vi "Vision Research Phantom Series PhFile Error Handler.vi"(0 "Error Code (0)":i32, 5 "Error In (no error)":errorcluster) -> (19 "Error Out":errorcluster)   [LabVIEW 2013, in "VRI.lvlib"]
doc: "This VI calls the PhGetErrorMessage funciton prototype for the PhFile.dll associated with the Vision Research Phantom Series cameras. An error message is created if an error code is returned.\n\nPlace this VI after any PhFile.dll call"
uses:
  VRI.lvlib
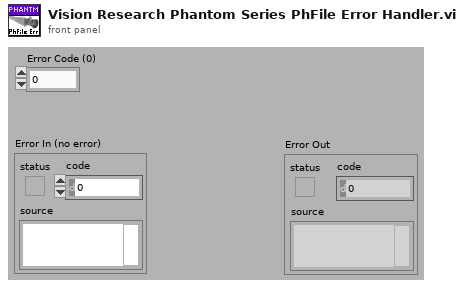
[diagram p1: front panel]
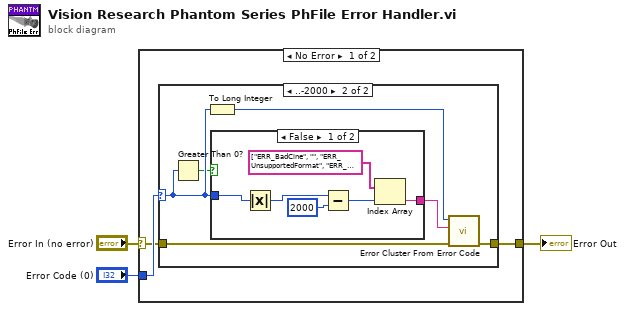
[diagram p0: block diagram]
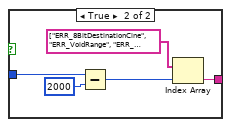
[diagram p3: hidden frame]
diagram:
  n1 = case shown="No Error" "Error In (no error)" {
    selector: "Error In (no error)" -> [w4 w25]
    tunnel: [w6 w25] -> w3
    tunnel: "Error Code (0)" -> [w5 _]
    frame No Error {
      n2 = case shown="..-2000" w5 {
        selector: w5 -> [_ w13]
        tunnel: w4 -> [w7 w11]
        tunnel: [w7 w10] -> w6
        frame 0, Default {
        }
        frame ..-2000 {
          n3 = Greater Than 0?(x=w13) -> (x > 0?=w12:bool)
          n4 = To Long Integer(number=w13) -> (32bit integer=w8:i32)
          n5 = case shown="False" w12 {
            tunnel: [w19 w24] -> w9
            tunnel: w13 -> [w15 w20]
            frame False {
              n6 = Absolute Value(x=w15) -> (abs(x)=w16:i32)
              n7 = Subtract(x=w16, y=2000) -> (x-y=w14:i32)
              n8 = Index Array(array=string[] ["ERR_BadCine", "", "ERR_UnsupportedFormat", "ERR_InsufficientAlloc", "ERR_NotInRange", "ERR_SaveAvi", "ERR_Encoder", "ERR_UnsupportedTiffFormat", "", "SplitQuartersUnsupported", "ERR_NotACineFile", "", "ERR_FileOpen", "ERR_FileRead", "ERR_FileWrite", "ERR_FileSeek", "ERR_DecompressImage", "ERR_CineVerNewer", "ERR_NotSupported", "", "", "ERR_CannotBuildGraph", "", "ERR_AuxDataNotFound", "ERR_NotEnoughMemory", "ERR_MpegReaderNotFound", "", "", "ERR_FunctionNotFound"], index=w14) -> (element=w19:string)
            }
            frame True {
              n9 = Subtract(x=w20, y=2000) -> (x-y=w21:i32)
              n10 = Index Array(array=string[] ["ERR_8BitDestinationCine", "ERR_VoidRange", "ERR_ReducedRange", "ERR_Seeking", "ERR_UserAbort", "ERR_FreeLibrary", "ERR_LeadToolsNotFound", "ERR_EVSNotFound"], index=w21) -> (element=w24:string)
            }
          }
          n11 = call <vilib>:"Error Cluster From Error Code.vi"("error in (no error)"=w11, "error message (\"\")"=w9, "error code (0)"=w8) -> ("error out"=w10:errorcluster)  [unwired: 6 in]
        }
      }
    }
    frame Error {
    }
  }
  "Error Out" <- w3
